vi "MEASURE_hysteresis.vi"() -> ()   [LabVIEW 2020]
uses:
  <vilib>/Utility/file.llb/Write To Spreadsheet File (DBL).vi
  <instrlib>/Stanford Research 830/Stanford Research 830.lvlib
  <instrlib>/Keithley 2450/Keithley 2450.lvlib
panel:
  out "loop run":i32
  in  "loop #":i32
  in  "Save data or not":bool=TRUE
  in  "path (folder + filename)":string="D:\\Kedar\\MoS2\\jw7_DJ_bulk_111213\\VvsHtr\\VvsHtr_300K"
  in  "Clear Plot":bool
  out "XY Graph":cluster{dbl[], dbl[]}(graph)
  out "LOCKIN Measurement":dbl
  in  "Parameter (1: X)":u16(ring)=1 items=["X"=1, "Y"=2, "R"=3, "Theta"=4, "Channel 1"=5, "Channel 2"=6, "Aux In 1"=7, "Aux In 2"=8, "Aux In 3"=9, "Aux In 4"=10]
  out "gate voltage":dbl format="%#_13g"
  out "gate leaking":string="defbuffer1"
  in  "GATE STEP(mv)":i32
  in  "GATE Low Value (default 0)":dbl=1.0
  in  "GATE High Value":dbl=1.0
  in  "Function (0: Volts) 2":u16(ring) items=["Volts", "Current", "Resistance"]
  in  "Source Compaliance":dbl=1e-06
  in  "V address":refnum<visa-resource-name>="GPIB0::24::INSTR"
  in  "SD stabilization(S) 2":dbl format="%#_13g"
  in  "Sine Output Amplitude (1 V) 2":dbl=1.0
  in  "GATE / SD stablization 3":dbl format="%#_13g"
  in  "frequency":dbl format="%#_13g"
  in  "Input Connection (0: Single-Ended Voltage)":u16(ring) items=["Single-Ended Voltage", "Differential Voltage", "1 MOhm Current Gain", "100 MOhm Current Gain"]
  in  "LOCKIN address":refnum<visa-resource-name>="GPIB0::24::INSTR"
  # "Lock-in"
  # "Gate Setting"
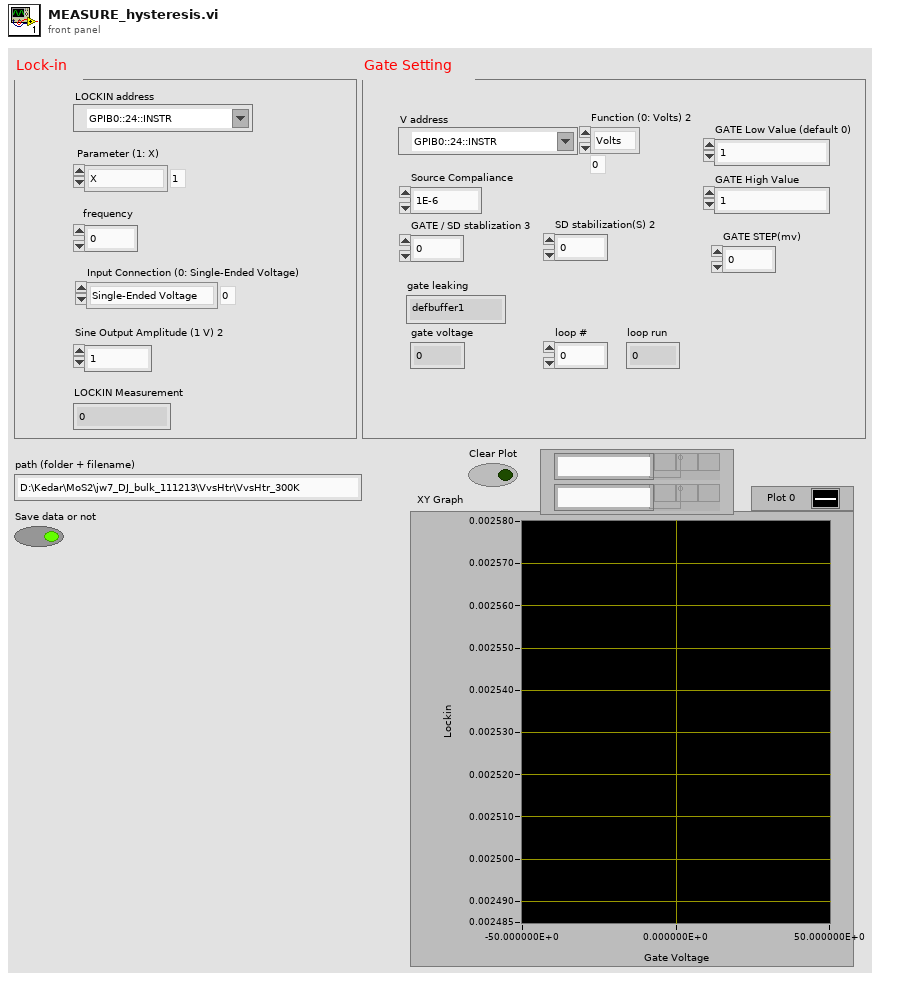
[diagram p1: front panel]
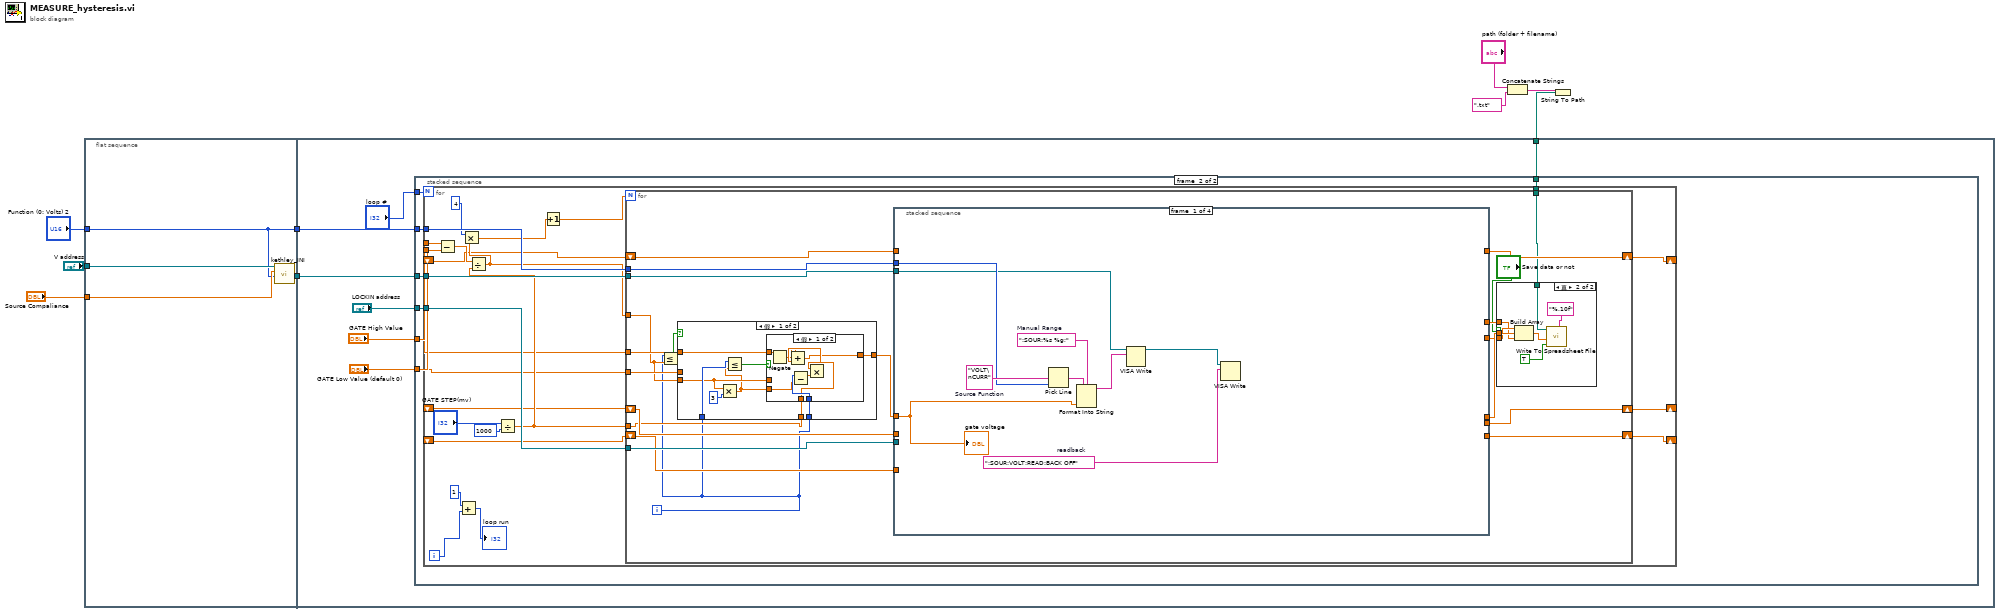
[diagram p0: block diagram]
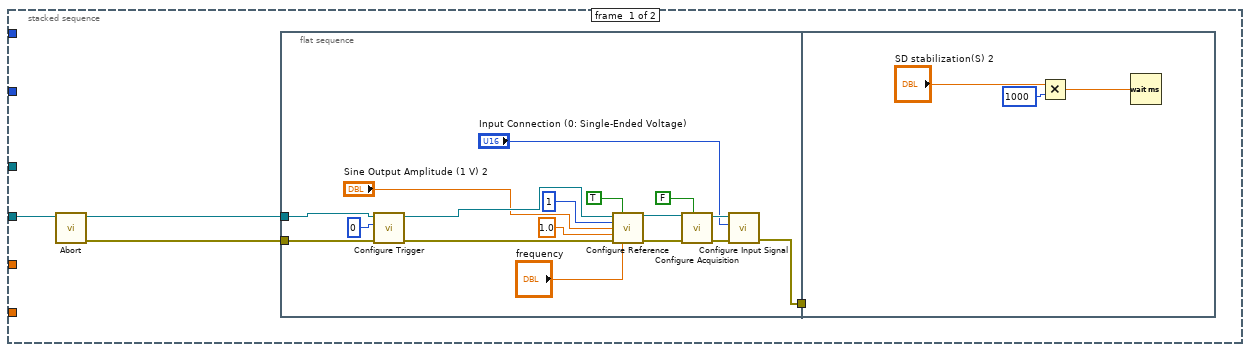
[diagram p2: hidden frame]
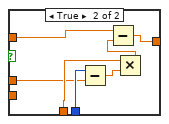
[diagram p4: hidden frame]
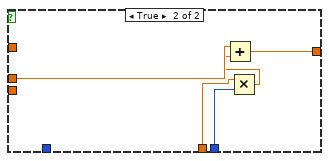
[diagram p5: hidden frame]
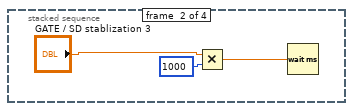
[diagram p6: hidden frame]
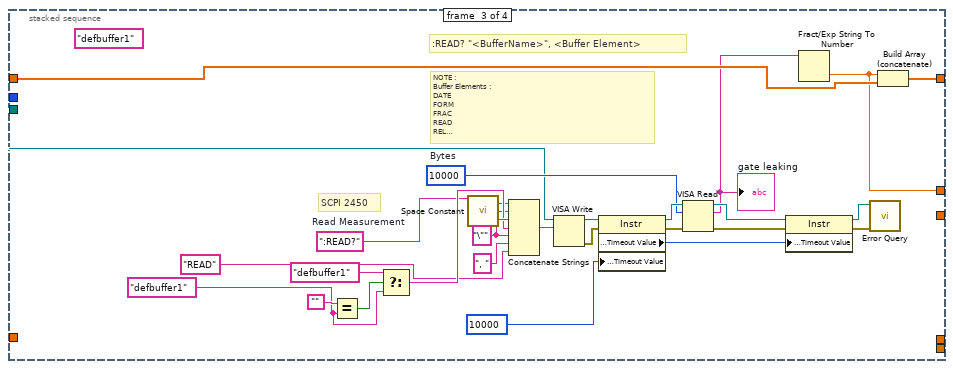
[diagram p7: hidden frame]
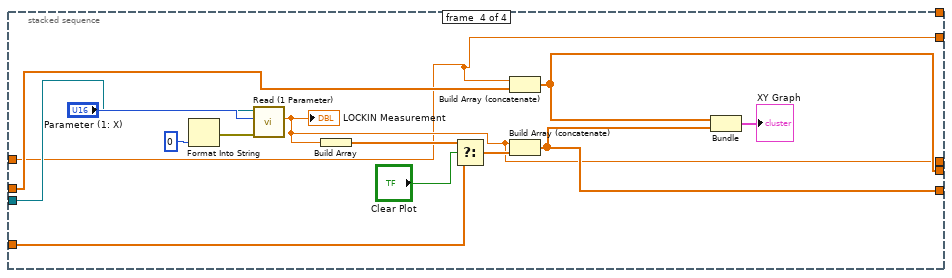
[diagram p8: hidden frame]
diagram:
  n1 = flat-sequence {
    tunnel: "V address" -> [w13]
    tunnel: "Source Compaliance" -> [w12]
    tunnel: "Function (0: Volts) 2" -> [w10]
    tunnel: [w11] -> w6
    tunnel: [w10] -> w5
    tunnel: w6 -> [w19]
    tunnel: w5 -> [w18]
    tunnel: w1 -> [w15]
    frame #0 {
      n2 = call "kethley_INI.vi"("Function (0: Volts) in"=w10, "Source Compaliance"=w12, "VISA Refnum in"=w13) -> ("VISA resource name out"=w11:refnum<visa-resource-name>)  [unwired: 8 in]
    }
    frame #1 {
      n3 = stacked-sequence {
        tunnel: "LOCKIN address" -> [w23 w49]
        tunnel: w19 -> [_ w50]
        tunnel: w18 -> [_ w51]
        tunnel: "GATE High Value" -> [_ w47]
        tunnel: "GATE Low Value (default 0)" -> [_ w48]
        tunnel: w15 -> [_ w46]
        tunnel: "loop #" -> [_ w45]
        frame #0 {
          n4 = call <instrlib>:"Abort.vi"("VISA resource name"=w23) -> ("error out"=w21:errorcluster, "VISA resource name out"=w22:refnum<visa-resource-name>)  [unwired: 9 in]
          n5 = flat-sequence {
            tunnel: w22 -> [w41]
            tunnel: [w26] -> w24
            tunnel: w21 -> [w25]
            tunnel: w24 -> [_]
            frame #0 {
              n6 = call <instrlib>:"Configure Trigger.vi"("error in (no error)"=w25, "Trigger Source (0: Internal)"=0, "VISA resource name"=w41) -> ("error out"=w35:errorcluster, "VISA resource name out"=w36:refnum<visa-resource-name>)  [unwired: 7 in]
              n7 = call <instrlib>:"Configure Reference.vi"("VISA resource name"=w36, "Auto Phase (T: Enabled)"=TRUE, "Reference Source (1: Internal)"=1, "Sine Output Amplitude (1 V)"="Sine Output Amplitude (1 V) 2", "Detection Harmonic Number (1)"=1.0 ("output voltage 2"), "error in (no error)"=w35, "Internal Reference Frequency (1000 Hz)"="frequency") -> ("VISA resource name out"=w33:refnum<visa-resource-name>, "error out"=w28:errorcluster)  [unwired: 7 in]
              n8 = call <instrlib>:"Configure Acquisition.vi"("Continuous Storage (T: Enable)"=FALSE, "error in (no error)"=w28, "VISA resource name"=w33) -> ("error out"=w27:errorcluster, "VISA resource name out"=w31:refnum<visa-resource-name>)  [unwired: 7 in]
              n9 = call <instrlib>:"Configure Input Signal.vi"("error in (no error)"=w27, "Input Connection (0: Single-Ended Voltage)"="Input Connection (0: Single-Ended Voltage)", "VISA resource name"=w31) -> ("error out"=w26:errorcluster)  [unwired: 7 in, 1 out]
            }
            frame #1 {
              n10 = Multiply(x="SD stabilization(S) 2", y=1000) -> (x*y=w44:dbl)
              n11 = Wait (ms)(milliseconds to wait=w44) -> ()  [unwired: 1 out]
            }
          }
        }
        frame #1 {
          n12 = for {
            N: w45 -> [_]
            tunnel: w51 -> [w74]
            tunnel: w50 -> [w73]
            tunnel: w49 -> [w72]
            tunnel: w48 -> [w66]
            tunnel: w47 -> [w65]
            tunnel: w46 -> [w64]
            shift-right: [w60] -> _
            shift-left: _ -> [w59]
            shift-right: [w58] -> _
            shift-left: _ -> [w56]
            shift-right: [w57] -> _
            shift-left: _ -> [w55]
            i -> [w53]
            n13 = Subtract(x=w65, y=w66) -> (x-y=w68:dbl)
            n14 = Add(x=1, y=w53) -> (x+y=→"loop run":i32)
            n15 = Divide(x="GATE STEP(mv)", y=1000) -> (x/y=w67:dbl)
            n16 = Divide(x=w68, y=w67) -> (x/y=w63:dbl)
            n17 = Multiply(x=4, y=w63) -> (x*y=w62:dbl)
            n18 = Increment(x=w62) -> (x+1=w61:dbl)
            n19 = for {
              N: w61 -> [_]
              tunnel: w74 -> [w95]
              tunnel: w73 -> [w94]
              tunnel: w72 -> [w93]
              tunnel: w67 -> [w84]
              shift-right: [w92] -> w60
              shift-left: w59 -> [w91]
              shift-right: [w88] -> w57
              shift-left: w55 -> [w90]
              shift-right: [w87] -> w58
              shift-left: w56 -> [w89]
              tunnel: w63 -> [w81]
              tunnel: w66 -> [w85]
              tunnel: w65 -> [w82]
              tunnel: w64 -> [w76]
              i -> [w80]
              n20 = Less Or Equal?(x=w80, y=w81) -> (x <= y?=w86:bool)
              n21 = case shown="假" w86 {
                tunnel: w85 -> [_ w131]
                tunnel: w80 -> [w111 w130]
                tunnel: w84 -> [w110 w129]
                tunnel: [w108 w127] -> w83
                tunnel: w82 -> [w109 _]
                tunnel: w81 -> [w104 _]
                tunnel: w80 -> [w107 _]
                frame False {
                  n22 = Multiply(x=w104, y=3) -> (x*y=w103:dbl)
                  n23 = Less Or Equal?(x=w107, y=w103) -> (x <= y?=w105:bool)
                  n24 = case shown="假" w105 {
                    tunnel: w111 -> [w119 w126]
                    tunnel: w110 -> [w117 w124]
                    tunnel: w109 -> [w113 w122]
                    tunnel: [w115 w121] -> w108
                    tunnel: w104 -> [_ w120]
                    tunnel: w103 -> [w112 _]
                    frame False {
                      n25 = Negate(x=w113) -> (-x=w114:dbl)
                      n26 = Subtract(x=w119, y=w112) -> (x-y=w118:dbl)
                      n27 = Multiply(x=w117, y=w118) -> (x*y=w116:dbl)
                      n28 = Add(x=w114, y=w116) -> (x+y=w115:dbl)
                    }
                    frame True {
                      n29 = Subtract(x=w126, y=w120) -> (x-y=w125:dbl)
                      n30 = Multiply(x=w124, y=w125) -> (x*y=w123:dbl)
                      n31 = Subtract(x=w122, y=w123) -> (x-y=w121:dbl)
                    }
                  }
                }
                frame True {
                  n32 = Multiply(x=w129, y=w130) -> (x*y=w128:dbl)
                  n33 = Add(x=w131, y=w128) -> (x+y=w127:dbl)
                }
              }
              n34 = stacked-sequence {
                tunnel: w95 -> [w136 _ _ _]
                tunnel: w94 -> [w135 _ w148 _]
                tunnel: w93 -> [_ _ _ w173]
                tunnel: w83 -> [w134 _ _ w171]
                tunnel: [_ _ w146 _] -> w92
                tunnel: w91 -> [_ _ w147 _]
                tunnel: w90 -> [_ _ _ w177]
                tunnel: w89 -> [_ _ _ w174]
                tunnel: [_ _ _ w176] -> w88
                tunnel: [_ _ _ w175] -> w87
                tunnel: [_ _ _ w172] -> w79
                tunnel: [_ _ _ w171] -> w78
                tunnel: [_ _ w144 _] -> w77
                frame #0 {
                  w132 = ":SOUR:VOLT:READ:BACK OFF"  # readback
                  w138 = "VOLT\nCURR"  # Source Function
                  w139 = ":SOUR:%s %g;"  # Manual Range
                  n35 = Pick Line(multi-line string=w138, line index=w136) -> (output string=w137:string)  [unwired: 1 out]
                  n36 = Format Into String(format string=w139, w137, w134) -> (resulting string=w140:string)  [unwired: 2 in, 1 out]
                  n37 = VISA Write(VISA resource name=w135, write buffer=w140) -> (VISA resource name out=w133:refnum<visa-resource-name>)  [unwired: 1 in, 2 out]
                  n38 = VISA Write(VISA resource name=w133, write buffer=w132) -> ()  [unwired: 1 in, 3 out]
                  "gate voltage" <- w134
                }
                frame #1 {
                  n39 = Multiply(x="GATE / SD stablization 3", y=1000) -> (x*y=w143:dbl)
                  n40 = Wait (ms)(milliseconds to wait=w143) -> ()  [unwired: 1 out]
                }
                frame #2 {
                  w159 = "defbuffer1" ("Buffer Name (defbuffer1) 2")
                  (unwired) "defbuffer1" ("t")
                  w157 = "\""
                  w154 = ":READ?"  # Read Measurement
                  w163 = u32 10000  # Bytes
                  # "NOTE :\nBuffer Elements :\nDATE\nFORM\nFRAC\nREAD\nREL\nSEC\nSOUR\nSOURFORM\nSOURSTAT\nSOURUNIT\nSTAT\nTIME\nTsT\nUNIT"
                  # ":READ? \"<BufferName>\", <Buffer Element>"
                  # "SCPI 2450"
                  n41 = Equal?(x="", y=w159) -> (x = y?=w160:bool)
                  n42 = Select(t="defbuffer1", s=w160, f=w159) -> (s? t:f=w156:string)
                  n43 = call <vilib>:"Space Constant.vi"() -> ("String"=w155:string)
                  n44 = Concatenate Strings(w154, w155, w157, w156, w157, ", " ("string"), "READ" ("Buffer Elements 2")) -> (w170:string)
                  n45 = VISA Write(VISA resource name=w148, write buffer=w170) -> (VISA resource name out=w162:refnum<visa-resource-name>, error out=w169:errorcluster)  [unwired: 1 in, 1 out]
                  n46 = property class="Instr"(reference=w162, error in=w169, "General Settings:Timeout Value"=10000 ("Timeout (10000 ms) 2")) -> (reference out=w168:refnum<visa-resource-name>, error out=w167:errorcluster, "General Settings:Timeout Value"=w164:u32)
                  n47 = VISA Read(VISA resource name=w168, byte count=w163, error in (no error)=w167) -> (VISA resource name out=w166:refnum<visa-resource-name>, read buffer=w145:string, error out=w165:errorcluster)  [unwired: 1 out]
                  "gate leaking" <- w145
                  n48 = property class="Instr"(reference=w166, error in=w165, "General Settings:Timeout Value"=w164) -> (reference out=w152:refnum<visa-resource-name>, error out=w151:errorcluster)
                  n49 = Fract/Exp String To Number(string=w145) -> (number=w144:dbl)  [unwired: 3 in, 1 out]
                  n50 = call <instrlib>:"Error Query.vi"("error in (no error)"=w151, "VISA resource name"=w152) -> ()  [unwired: 10 out]
                  n51 = Build Array (concatenate)(w144, w147) -> (w146:dbl[])
                }
                frame #3 {
                  n52 = Format Into String(0) -> (error out=w184:errorcluster)  [unwired: 3 in, 1 out]
                  n53 = call <instrlib>:"Read (1 Parameter).vi"("error in (no error)"=w184, "Parameter (1: X)"="Parameter (1: X)", "VISA resource name"=w173) -> ("Measurement"=w172:dbl)  [unwired: 6 in, 2 out]
                  "LOCKIN Measurement" <- w172
                  n54 = Build Array(w172) -> (w181:dbl[])
                  n55 = Select(t=w181, s="Clear Plot", f=w177) -> (s? t:f=w182:dbl[])
                  n56 = Build Array (concatenate)(w171, w174) -> (w175:dbl[])
                  n57 = Build Array (concatenate)(w172, w182) -> (w176:dbl[])
                  n58 = Bundle(w175, w176) -> (→"XY Graph":cluster{dbl[], dbl[]})  [unwired: 1 in]
                }
              }
              n59 = case shown="真" "Save data or not" {
                tunnel: w79 -> [_ w102]
                tunnel: w78 -> [_ w101]
                tunnel: w77 -> [_ w100]
                tunnel: w76 -> [_ w98]
                frame False {
                }
                frame True {
                  n60 = Build Array(w101, w102, w100) -> (w99:dbl[])
                  n61 = call-poly <vilib>:"Write To Spreadsheet File.vi"("format (%.3f)"="%.10f", "append to file? (new file:F)"=TRUE, "1D data"=w99, "file path (dialog if empty)"=w98) -> ()  [unwired: 4 in, 1 out]
                }
              }
            }
          }
        }
      }
    }
  }
  n62 = Concatenate Strings("path (folder + filename)", ".txt") -> (w2:string)
  n63 = String To Path(string=w2) -> (path=w1:path)
